vi "AddClassProperties.vi"(9 "Count":i32, 11 "Math.lvclass":refnum<class "Math.lvclass">) -> (3 "Math.lvclass 2":refnum<class "Math.lvclass">)   [LabVIEW 2016, in "Math.lvclass"]
uses:
  Math.lvclass
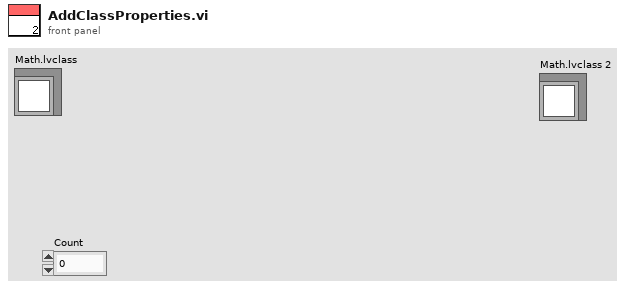
[diagram p1: front panel]
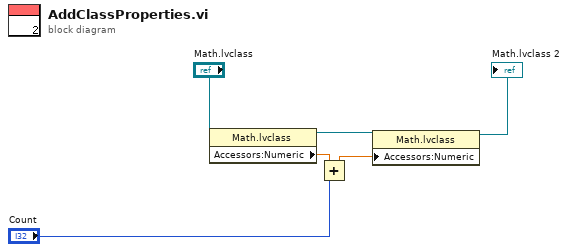
[diagram p0: block diagram]
diagram:
  n1 = property class="Math.lvclass"(reference="Math.lvclass") -> (reference out=w5:refnum<class "Math.lvclass">, "Accessors:Numeric"=w4:dbl)  [unwired: 1 in, 1 out]
  n2 = Add(x=w4, y="Count") -> (x+y=w2:dbl)
  n3 = property class="Math.lvclass"(reference=w5, "Accessors:Numeric"=w2) -> (reference out=→"Math.lvclass 2":refnum<class "Math.lvclass">)  [unwired: 1 in, 1 out]
